vi "PianoTest 1 channel.vi"() -> ()   [LabVIEW 2013]
uses:
  <vilib>/rvi/Emulation/niFpgaSctlEmulationGetInTimedLoop.vi
  <vilib>/rvi/Emulation/niFpgaEmulationReportErrorSimple.vi
  <vilib>/rvi/Emulation/niFpgaGetClockAttributes.vi
  <vilib>/rvi/eio/common/nirviEmuTemplateMethod_errors.vi
  <vilib>/rvi/Emulation/niFpgaCriticalErrorInLSC.vi
  <vilib>/rvi/FXPMathLib/FxpMul/XNode/nifxpmath_Multiplier.xnode
  <vilib>/rvi/FXPMathLib/FxpSub/XNode/nifxpmath_Sub.xnode
  <vilib>/eio/EIONode/EIONode.xnode
  <vilib>/rvi/FXPMathLib/sim/FxpSim.dll
panel:
  in  "PWM1 Duty Cycle %":fxp<+/-,20,16>
  in  "PWM1 Period (us)":fxp<+/-,20,16>
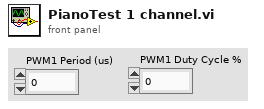
[diagram p1: front panel]
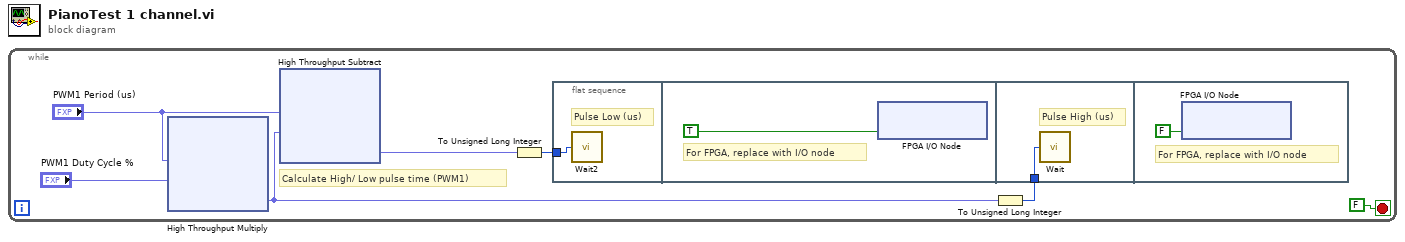
[diagram p0: block diagram]
diagram:
  n1 = while {
    stop <- FALSE stop-if-true
    # "Calculate High/ Low pulse time (PWM1)"
    n2 = xnode "High Throughput Multiply"("x"="PWM1 Period (us)", "y"="PWM1 Duty Cycle %") -> ("x*y"=w2:fxp<+/-,40,32>)
    n3 = xnode "High Throughput Subtract"("x"="PWM1 Period (us)", "y"=w2) -> ("x-y"=w1:fxp<+/-,41,33>)
    n4 = To Unsigned Long Integer(number=w1) -> (unsigned 32bit integer=w6:u32)
    n5 = flat-sequence {
      tunnel: w6 -> [w8]
      tunnel: w7 -> [w10]
      frame #0 {
        # "Pulse Low (us)"
        n6 = call "Wait2"("Count(uSec)"=w8) -> ()  [unwired: 1 out]
      }
      frame #1 {
        # "For FPGA, replace with I/O node"
        n7 = xnode "FPGA I/O Node"("Mod1/DO0"=TRUE ("PWM 1T")) -> ()  [unwired: 1 in, 1 out]
      }
      frame #2 {
        # "Pulse High (us)"
        n8 = call "Wait"("Count(uSec)"=w10) -> ()  [unwired: 1 out]
      }
      frame #3 {
        # "For FPGA, replace with I/O node"
        n9 = xnode "FPGA I/O Node"("Mod1/DO0"=FALSE ("PWM 1T")) -> ()  [unwired: 1 in, 1 out]
      }
    }
    n10 = To Unsigned Long Integer(number=w2) -> (unsigned 32bit integer=w7:u32)
  }
